vi "Example 3 - Multiple Buses Multiple Types.vi"() -> ()   [LabVIEW 2021]
uses:
  Omni-Bus/Omni_Bus.lvclass
  Omni-Bus/Support/Broad Types.ctl
  Local Bus/Local Bus.lvclass
  C:/Users/Tim/Documents/GitHub/Omni-Bus/Source/Omni-Bus/Bus Access/Bus_Access.lvclass
  <vilib>/Utility/Data Type/Type Definitions/Data Type.ctl
  Aggregator Bus/Aggregator Bus.lvclass
  Omni-Bus/Support/Read/Read DBL.vi
  Omni-Bus/Support/Read/Read String.vi
  Omni-Bus/Support/Read/Read Boolean.vi
  Omni-Bus/Support/Read/Read Time.vi
  <vilib>/TSA/Abstract Data Classes/Constants/Support/DBL/Const_DBL.lvclass
  C:/Program Files (x86)/National Instruments/LabVIEW 2021/vi.lib/TSA/Abstract Data Classes/Abs_Types/Numeric/Abs_Numeric.lvclass
  <vilib>/TSA/Abstract Data Classes/Abs_Types/Time/Abs_Time.lvclass
  <vilib>/TSA/Abstract Data Classes/Abs_Types/Numeric/Abs_Numeric.lvclass
  C:/Program Files (x86)/National Instruments/LabVIEW 2021/vi.lib/TSA/Abstract Data Classes/Abs_Types/Type/Abs_Type.lvclass
  <vilib>/TSA/Abstract Data Classes/Abs_Types/Double Float/Abs_Double Float.lvclass
  <vilib>/TSA/Abstract Data Classes/Abs_Types/String/Abs_String.lvclass
  <vilib>/TSA/Abstract Data Classes/Abs_Types/Boolean/Abs_Boolean.lvclass
  <vilib>/TSA/Abstract Data Classes/Constants/Support/DBL/DBL.vi
  Omni-Bus/Support/Write/Write Boolean.vi
  Omni-Bus/Support/Write/Write String.vi
  Omni-Bus/Support/Write/Write DBL.vi
  <vilib>/Utility/Data Type/NI_Data Type.lvlib
panel:
  out "Read Time Error":errorcluster
  out "Time Stamp":timestamp
  in  "Read Time Tag":string
  in  "Write Boolean Tag":string
  in  "Boolean":bool
  out "Write Boolean error":errorcluster
  in  "Write String Tag":string
  in  "String":string
  out "Write String error":errorcluster
  out "Read Bool Error":errorcluster
  out "Read String error":errorcluster
  out "Boolean":bool
  out "String":string
  in  "Read Bool Tag":string
  in  "Read String Tag":string
  out "Read DBL error":errorcluster
  out "Write DBL error":errorcluster
  in  "Double":dbl
  in  "Write DBL Tag":string
  in  "stop":bool
  out "Double":dbl format="%.2f"
  in  "Read DBL Tag":string
  out "error out":errorcluster
  out "All Tags":string[](array[string])
  # "The advantage of the \nOmni-bus is its ability \nto aggregate other\ndata storage and IO\nbus systems.\nMore options will become \navailable as they are developed."
  # "The Aggregator Bus Class\ncan combine other classes\nthat conform to the other\nTSA LV Abstract Data Types"
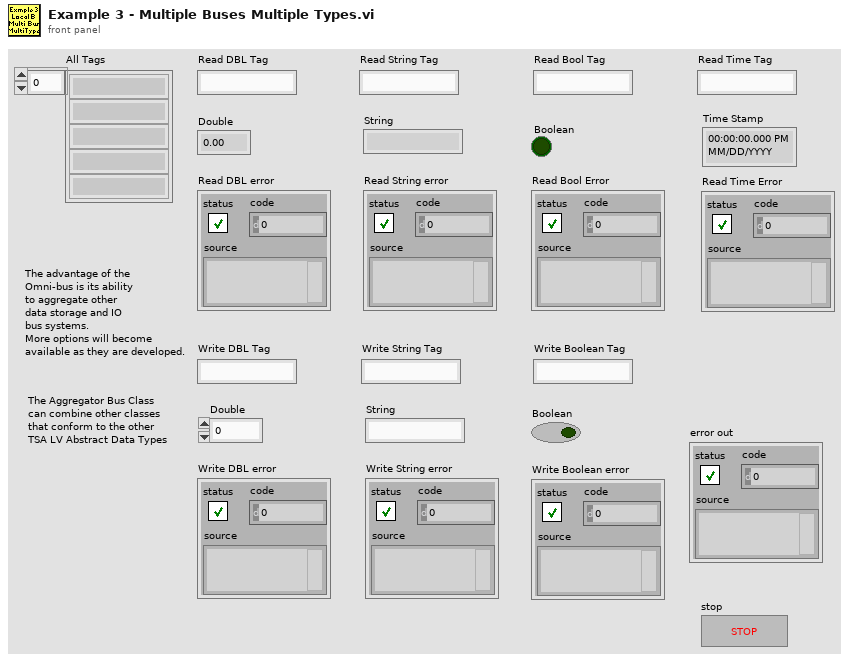
[diagram p1: front panel]
types:
  T1 = typedef "NI_Data Type.lvlib/Data Type.ctl" = enum8{"Invalid Type", "Void", "I8", "I16", "I32", "I64", "U8", "U16", "U32", "U64", "Single Float", "Double Float", "Extended Float", "Single Complex", "Double Complex", "Extended Complex", "Enum U8", "Enum U16", "Enum U32", "Enum U64", "Single Float With Unit", "Double Float With Unit", "Extended Float With Unit", "Single Complex with Unit", "Double Complex with Unit", "Extended Complex with Unit", "Boolean", "String", "Path", "Picture", "Tag", "Array", "Cluster", "Variant", "LV Variant", "Waveform", "Timestamp", "Digital Waveform", "Digital Data", "ExpressData", "Refnum", "External Data", "VI", "Poly VI", "LabVIEW Class Instance", "Fixed Point", "Set Collection", "Map Collection"}
  T2 = typedef "Omni_Bus.lvclass/Broad Types.ctl" = enum16{"All Tags", "NI Specific Type", "Boolean", "String", "Numeric", "Float", "Integer", "Collection", "All Value Types", "Non Value Types"}
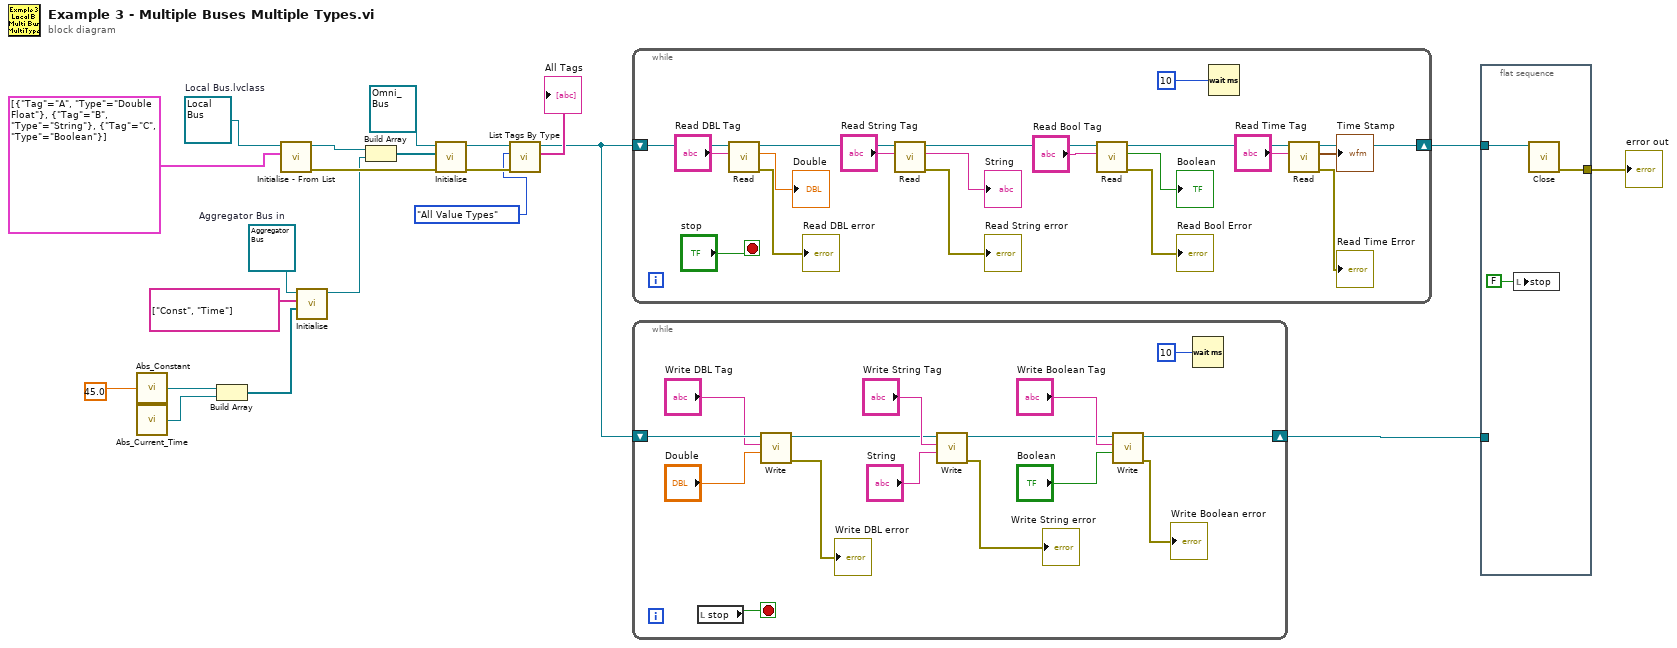
[diagram p0: block diagram]
diagram:
  w6 = refnum<class "Aggregator Bus.lvclass"> refnum  # Aggregator Bus in
  w9 = refnum<class "Local Bus.lvclass"> refnum  # Local Bus.lvclass
  n1 = call-poly <vilib>:"Abs_Constant.vi"("Value"=45.0) -> ("Constant"=w4:refnum<class "Const_DBL.lvclass">)  [unwired: 4 in]
  n2 = call <vilib>:"Abs_Current_Time.vi"() -> ("Abs_Time.lvclass"=w2:refnum<class "Abs_Time.lvclass">)  [unwired: 5 in]
  n3 = Build Array(w4, w2) -> (w3:refnum<class "Abs_Numeric.lvclass">[])
  n4 = call "Initialise - From List.vi"("Tag List"=cluster{"Tag":string, "Type":T1}[] [{"Tag"="A", "Type"=enum."Double Float"}, {"Tag"="B", "Type"=enum."String"}, {"Tag"="C", "Type"=enum."Boolean"}], "Local Bus in"=w9) -> ("error out"=w11:errorcluster, "Local Bus out"=w10:refnum<class "Local Bus.lvclass">)  [unwired: 8 in]
  n5 = call "Initialise.vi"("Values"=w3, "Tags"=string[] ["Const", "Time"], "Aggregator Bus in"=w6) -> ("Aggregator Bus out"=w7:refnum<class "Aggregator Bus.lvclass">)  [unwired: 7 in, 1 out]
  n6 = Build Array(w10, w7) -> (w20:refnum<class "Bus_Access.lvclass">[])
  n7 = call-dynamic "Initialise.vi"("error in (no error)"=w11, "Bus Access"=w20, "Var Bus in"=refnum<class "Omni_Bus.lvclass"> refnum) -> ("error out"=w18:errorcluster, "Var Bus out"=w19:refnum<class "Omni_Bus.lvclass">)  [unwired: 7 in]
  n8 = call-dynamic "List Tags By Type.vi"("error in (no error)"=w18, "Broad Types"=Broad_Types."All Value Types", "Var Bus in"=w19) -> ("Tags"=→"All Tags":string[], "Var Bus out"=w13:refnum<class "Omni_Bus.lvclass">)  [unwired: 5 in, 2 out]
  n9 = while {
    shift-right: [w25] -> w14
    shift-left: w13 -> [w40]
    stop <- "stop" stop-if-true
    n10 = call-poly "Read.vi"("Tag"="Read DBL Tag", "Var Bus in"=w40) -> ("error out"=→"Read DBL error":errorcluster, "Numeric"=→"Double":dbl, "Var Bus out"=w33:refnum<class "Omni_Bus.lvclass">)  [unwired: 7 in]
    n11 = call-poly "Read.vi"("Tag"="Read String Tag", "Var Bus in"=w33) -> ("error out"=→"Read String error":errorcluster, "String"=→"String":string, "Var Bus out"=w31:refnum<class "Omni_Bus.lvclass">)  [unwired: 7 in]
    n12 = call-poly "Read.vi"("Tag"="Read Bool Tag", "Var Bus in"=w31) -> ("error out"=→"Read Bool Error":errorcluster, "Boolean"=→"Boolean":bool, "Var Bus out"=w26:refnum<class "Omni_Bus.lvclass">)  [unwired: 7 in]
    n13 = Wait (ms)(milliseconds to wait=u32 10) -> ()  [unwired: 1 out]
    n14 = call-poly "Read.vi"("Tag"="Read Time Tag", "Var Bus in"=w26) -> ("error out"=→"Read Time Error":errorcluster, "Time Stamp"=→"Time Stamp":timestamp, "Var Bus out"=w25:refnum<class "Omni_Bus.lvclass">)  [unwired: 7 in]
  }
  n15 = while {
    shift-right: [w41] -> w12
    shift-left: w13 -> [w55]
    stop <- w52 stop-if-true
    n16 = local read "stop"() -> (w52:bool)
    n17 = call-poly "Write.vi"("Numeric"="Double", "Tag"="Write DBL Tag", "Omni_Bus in"=w55) -> ("error out"=→"Write DBL error":errorcluster, "Omni_Bus out"=w46:refnum<class "Omni_Bus.lvclass">)  [unwired: 7 in]
    n18 = call-poly "Write.vi"("String"="String", "Tag"="Write String Tag", "Omni_Bus in"=w46) -> ("error out"=→"Write String error":errorcluster, "Omni_Bus out"=w42:refnum<class "Omni_Bus.lvclass">)  [unwired: 7 in]
    n19 = call-poly "Write.vi"("Boolean"="Boolean", "Tag"="Write Boolean Tag", "Omni_Bus in"=w42) -> ("error out"=→"Write Boolean error":errorcluster, "Omni_Bus out"=w41:refnum<class "Omni_Bus.lvclass">)  [unwired: 7 in]
    n20 = Wait (ms)(milliseconds to wait=u32 10) -> ()  [unwired: 1 out]
  }
  n21 = flat-sequence {
    tunnel: [w58] -> w15
    tunnel: w14 -> [w57]
    tunnel: w12 -> [_]
    frame #0 {
      n22 = local write "stop"(FALSE ("stop")) -> ()
      n23 = call-dynamic "Close.vi"("Data in"=w57) -> ("error out"=w58:errorcluster)  [unwired: 9 in, 1 out]
    }
  }
  "error out" <- w15
